vi "parse_Vector3Stamped.vi"(4 "error in":errorcluster, 7 "msg in":string) -> (0 "error out":errorcluster, 1 "Vector3":cluster{"x":dbl, "y":dbl, "z":dbl}, 2 "Header":T1, 3 "msg out":string)   [LabVIEW 2014]
doc: "Parses a message into a vector 3 stamped"
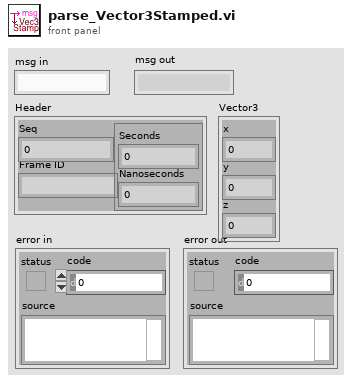
[diagram p1: front panel]
types:
  T1 = cluster{"Seq":u32, "Frame ID":string, "Timestamp":cluster{"Seconds":i32, "Nanoseconds":i32}}
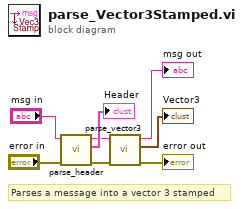
[diagram p0: block diagram]
diagram:
  # "Parses a message into a vector 3 stamped"
  n1 = call "parse_header.vi"("error in"="error in", "msg in"="msg in") -> ("error out"=w4:errorcluster, "Header"=→"Header":T1, "msg out"=w5:string)  [unwired: 3 in]
  n2 = call "parse_vector3.vi"("error in"=w4, "msg in"=w5) -> ("error out"=→"error out":errorcluster, "Vector3"=→"Vector3":cluster{"x":dbl, "y":dbl, "z":dbl}, "msg out"=→"msg out":string)  [unwired: 3 in]
